vi "JKI SM Helper Controls.vi"() -> ()   [LabVIEW 2020]
uses:
  btn-clear-history-36x36.ctl
  btn-forward-36x36.ctl
  btn-refresh-36x36.ctl
  btn-back-36x36.ctl
panel:
  in  "Back":T1
  in  "Refresh":T2
  in  "Forward":T3
  in  "Clear History":T4
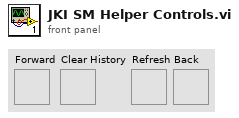
[diagram p1: front panel]
types:
  T1 = typedef "btn-back-36x36.ctl" = bool
  T2 = typedef "btn-refresh-36x36.ctl" = bool
  T3 = typedef "btn-forward-36x36.ctl" = bool
  T4 = typedef "btn-clear-history-36x36.ctl" = bool
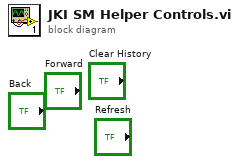
[diagram p0: block diagram]
diagram:
